vi "exponential histogram model.vi"(3 "output control":T1, 4 "data":variant, 5 "X":dbl[](array[numeric]), 6 "a":dbl[](array[numeric])) -> (0 "error out":errorcluster, 1 "f'(X,a)":dbl[][](array[numeric]), 2 "f(X,a)":dbl[](array[numeric]))   [LabVIEW 2017]
doc: "Sum of three Gaussians, plus DC offset."
uses:
  <vilib>/gmath/NumericalOptimization/LM_output select.ctl
  <vilib>/gmath/NI_Gmath.lvlib
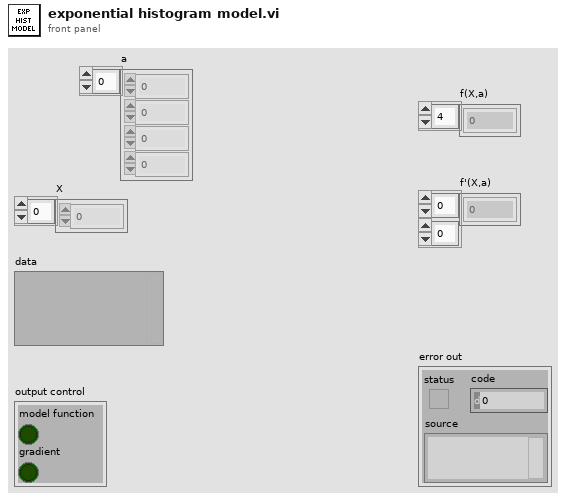
[diagram p1: front panel]
types:
  T1 = typedef "NI_Gmath.lvlib/LM_output select.ctl" = cluster{"model function":bool, "gradient":bool}
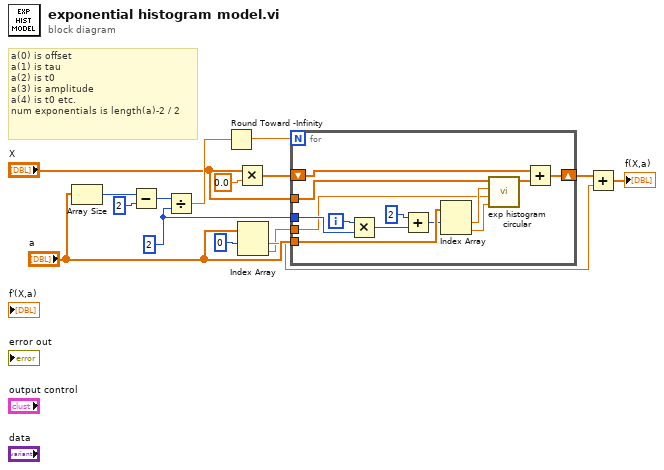
[diagram p0: block diagram]
diagram:
  w11 = 2 ("y")
  # "a(0) is offset\na(1) is tau\na(2) is t0\na(3) is amplitude\na(4) is t0 etc.\nnum exponentials is length(a)-2 / 2"
  n1 = Array Size(array="a") -> (size(s)=w15:i32)
  n2 = Subtract(x=w15, y=2 ("x")) -> (x-y=w14:i32)
  n3 = Divide(x=w14, y=w11) -> (x/y=w13:dbl)
  n4 = Round Toward -Infinity(1:w13) -> (0:w12:dbl)
  n5 = Multiply(x="X", y=0.0) -> (x*y=w8:dbl[])
  n6 = Index Array(array="a", index #1=0 ("index")) -> (element #1=w4:dbl, element #2=w2:dbl)  [unwired: 1 in]
  n7 = for {
    N: w12 -> [_]
    tunnel: "X" -> [w28]
    tunnel: "a" -> [w27]
    tunnel: w11 -> [w25]
    shift-right: [w20] -> w7
    shift-left: w8 -> [w21]
    tunnel: w2 -> [w18]
    i -> [w26]
    n8 = Multiply(x=w26, y=w25) -> (x*y=w24:i32)
    n9 = Add(x=2, y=w24) -> (x+y=w19:i32)
    n10 = Index Array(array=w27, index #1=w19) -> (element #1=w23:dbl, element #2=w16:dbl)  [unwired: 1 in]
    n11 = call "exp histogram circular.vi"("amplitude"=w16, "tau"=w18, "t0"=w23, "bin number"=w28) -> ("hist prediction"=w22:dbl[])  [unwired: 7 in]
    n12 = Add(x=w21, y=w22) -> (x+y=w20:dbl[])
  }
  n13 = Add(x=w7, y=w4) -> (x+y=→"f(X,a)":dbl[])
